vi "Do.vi"(8 "error in (no error)":errorcluster, 10 "Actor in":refnum<class "Actor.lvclass">, 11 "ConnectionClosed Msg":refnum<class "ConnectionClosed Msg.lvclass">) -> (0 "error out":errorcluster, 2 "Actor out":refnum<class "Actor.lvclass">)   [LabVIEW 2023, in "TCP_Server_Connection_Handler.lvlib" / "ConnectionClosed Msg.lvclass"]
doc: "This VI delivers the message to the actor by calling the appropriate method(s) on the actor."
uses:
  ConnectionClosed Msg.lvclass
  ConnectionClosed Msg.lvclass/ConnectionClosed Msg.ctl
  fe599be5-368c-4233-8e05-236c10db8dcc.vi
  TCP_Connections_Controller/TCP_Connections_Controller.lvclass
  <vilib>/ActorFramework/Actor/Actor.lvclass
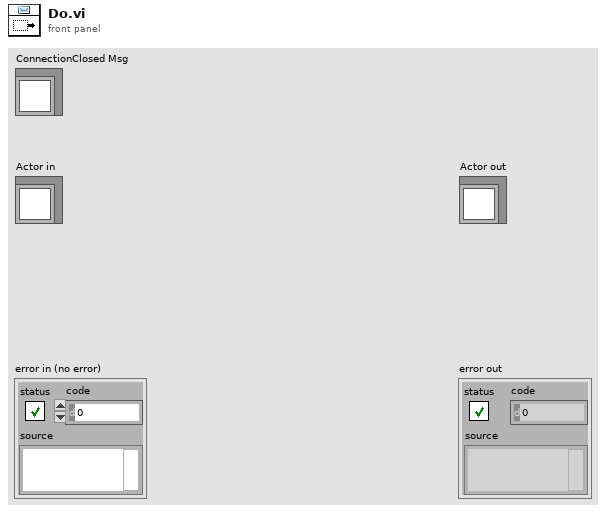
[diagram p1: front panel]
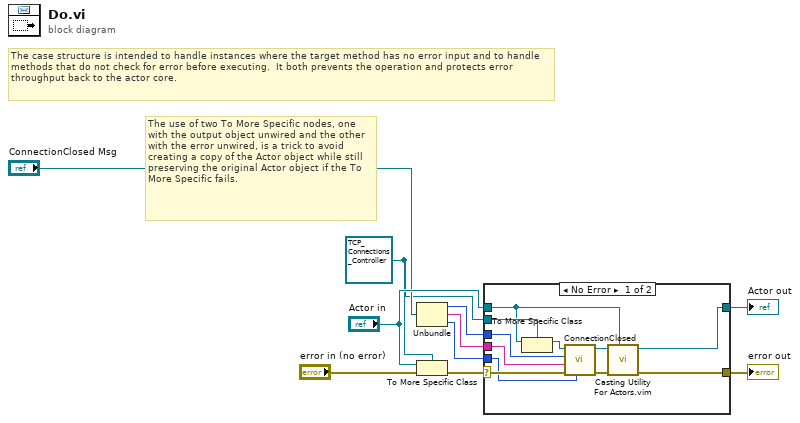
[diagram p0: block diagram]
diagram:
  w5 = refnum<class "TCP_Connections_Controller.lvclass"> refnum ("Actor in")
  # "The use of two To More Specific nodes, one with the output object unwired and the other with the error unwired, is a trick to avoid creating a copy of the Actor object while still preserving the original Actor object if the To More Specific fails."
  # "The case structure is intended to handle instances where the target method has no error input and to handle methods that do not check for error before executing.  It both prevents the operation and protects error throughput back to the actor core."
  n1 = Unbundle("ConnectionClosed Msg") -> (w3:i32, w2:string, w1:i32)
  n2 = To More Specific Class(target class=w5, reference="Actor in", error in="error in (no error)") -> (error out=w4:errorcluster)  [unwired: 1 out]
  n3 = case shown="No Error" w4 {
    selector: w4 -> [w21 w23]
    tunnel: [w15 w23] -> w10
    tunnel: [w16 w22] -> w9
    tunnel: "Actor in" -> [w18 w22]
    tunnel: w5 -> [w19 _]
    tunnel: w3 -> [w13 _]
    tunnel: w2 -> [w12 _]
    tunnel: w1 -> [w11 _]
    frame No Error {
      n4 = To More Specific Class(target class=w19, reference=w18) -> (specific class reference=w20:refnum<class "TCP_Connections_Controller.lvclass">)  [unwired: 1 in, 1 out]
      n5 = call-dynamic "ConnectionClosed.vi"("FinaErrorCode"=w11, "error in (no error)"=w21, "ClientIP"=w12, "ConnectionNumber"=w13, "TCP_Connections_Controller in"=w20) -> ("error out"=w14:errorcluster, "TCP_Connections_Controller out"=w17:refnum<class "TCP_Connections_Controller.lvclass">)  [unwired: 5 in]
      n6 = call "Casting Utility For Actors.vim"("type"=w18, "error in (no error)"=w14, "Actor in"=w17) -> ("error out"=w15:errorcluster, "Actor out"=w16:refnum<class "Actor.lvclass">)  [unwired: 7 in]
    }
    frame Error {
      # "If type check fails, pass the original object out again."
    }
  }
  "error out" <- w10
  "Actor out" <- w9
